vi "Init Queues.vi"(9 "Self-To-Caller":refnum<class "Message Enqueuer.lvclass">, 10 "Self-ToSelf":refnum<class "Message Priority Queue.lvclass">, 11 "Actor in":refnum<class "Actor.lvclass">) -> (3 "Actor out":refnum<class "Actor.lvclass">)   [LabVIEW 2017, in "Actor Framework.lvlib" / "Actor.lvclass"]
uses:
  <vilib>/ActorFramework/Actor/Actor.lvclass
  <vilib>/ActorFramework/Message Priority Queue/Message Priority Queue.lvclass
  <vilib>/ActorFramework/Message Enqueuer/Message Enqueuer.lvclass
  <vilib>/ActorFramework/Actor/Actor.lvclass/Actor.ctl
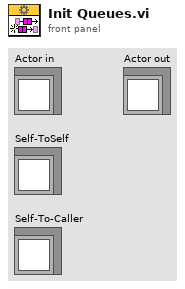
[diagram p1: front panel]
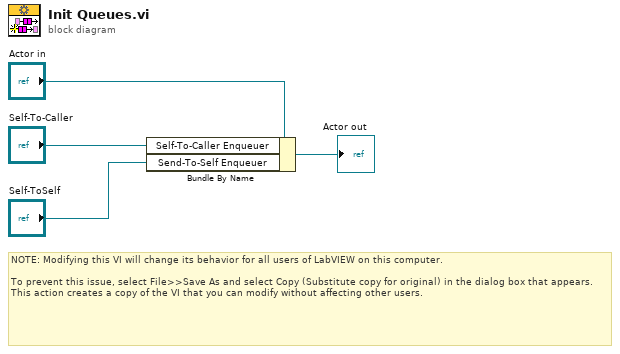
[diagram p0: block diagram]
diagram:
  # "NOTE: Modifying this VI will change its behavior for all users of LabVIEW on this computer.\n\nTo prevent this issue, select File>>Save As and select Copy (Substitute copy for original) in the dialog box that appears. This action creates a copy of the VI that you can modify without affecting other users."
  n1 = Bundle By Name(cluster="Actor in", "Self-To-Caller Enqueuer"="Self-To-Caller", "Send-To-Self Enqueuer"="Self-ToSelf") -> (→"Actor out":refnum<class "Actor.lvclass">)
